vi "Get Process Info.vi"(8 "error in (no error)":errorcluster, 11 "process handle":refnum<k24>) -> (0 "error out":errorcluster, 3 "process information":dbl[](array[numeric]))   [LabVIEW 2016]
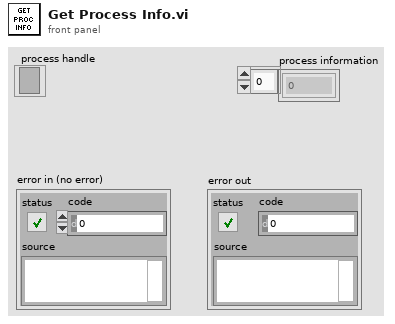
[diagram p1: front panel]
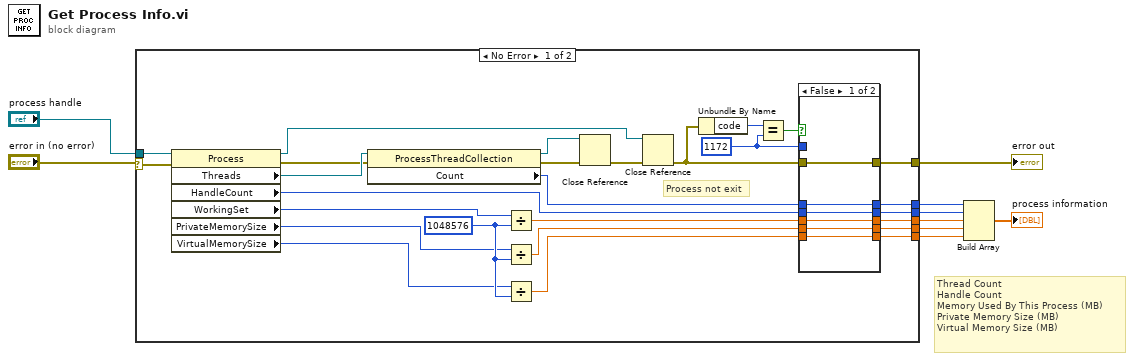
[diagram p0: block diagram]
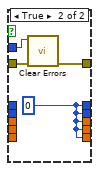
[diagram p2: hidden frame]
diagram:
  # "Thread Count\nHandle Count\nMemory Used By This Process (MB)\nPrivate Memory Size (MB)\nVirtual Memory Size (MB)"
  n1 = case shown="No Error" "error in (no error)" {
    selector: "error in (no error)" -> [w10 w47]
    tunnel: "process handle" -> [w26 _]
    tunnel: [w23 _] -> w8
    tunnel: [w21 _] -> w7
    tunnel: [w19 _] -> w6
    tunnel: [w17 _] -> w5
    tunnel: [w15 _] -> w4
    tunnel: [w13 w47] -> w2
    frame No Error {
      w11 = 1172 ("y")
      w36 = i64 1048576 ("y")
      # "Process not exit"
      n2 = property class="Process"(reference=w26, error in=w10) -> (reference out=w30:refnum<k24>, error out=w27:errorcluster, "Threads"=w32:refnum<k24>, "HandleCount"=w20:i32, "WorkingSet"=w33:i32, "PrivateMemorySize"=w34:i32, "VirtualMemorySize"=w35:i32)
      n3 = property class="ProcessThreadCollection"(reference=w32, error in=w27) -> (reference out=w28:refnum<k24>, error out=w29:errorcluster, "Count"=w22:i32)
      n4 = Divide(x=w33, y=w36) -> (x/y=w18:dbl)
      n5 = Divide(x=w34, y=w36) -> (x/y=w16:dbl)
      n6 = Divide(x=w35, y=w36) -> (x/y=w14:dbl)
      n7 = Close Reference(reference=w28, error in (no error)=w29) -> (error out=w31:errorcluster)
      n8 = Close Reference(reference=w30, error in (no error)=w31) -> (error out=w12:errorcluster)
      n9 = Unbundle By Name(w12) -> ("code"=w25:i32)
      n10 = Equal?(x=w25, y=w11) -> (x = y?=w24:bool)
      n11 = case shown="False" w24 {
        tunnel: [w41 w45] -> w23
        tunnel: w22 -> [w41 _]
        tunnel: [w40 w45] -> w21
        tunnel: w20 -> [w40 _]
        tunnel: [w39 w45] -> w19
        tunnel: w18 -> [w39 _]
        tunnel: [w38 w45] -> w17
        tunnel: w16 -> [w38 _]
        tunnel: [w37 w45] -> w15
        tunnel: w14 -> [w37 _]
        tunnel: [w42 w44] -> w13
        tunnel: w12 -> [w42 w46]
        tunnel: w11 -> [_ w43]
        frame False {
        }
        frame True {
          w45 = 0
          n12 = call <vilib>:"Clear Errors.vi"("error in (no error)"=w46, "specific error code to clear (0: all)"=w43) -> ("error out"=w44:errorcluster)  [unwired: 4 in, 1 out]
        }
      }
    }
    frame Error {
    }
  }
  "error out" <- w2
  n13 = Build Array(w8, w7, w6, w5, w4) -> (→"process information":dbl[])
